vi "Write DI-B Profiles.vi"(8 "error in (no error)":errorcluster, 10 "DI-B Profiles - Pulse Width [s]":sgl[][](array[numeric]), 11 "DCM-DSI-HW in":refnum<class "DCM-DSI.lvclass">) -> (0 "error out":errorcluster, 3 "DCM-DSI-HW out":refnum<class "DCM-DSI.lvclass">)   [LabVIEW 2016, in "DCM-DSI.lvclass"]
uses:
  DCM-DSI.lvclass
  DCM-DSI.lvclass/DCM-DSI.ctl
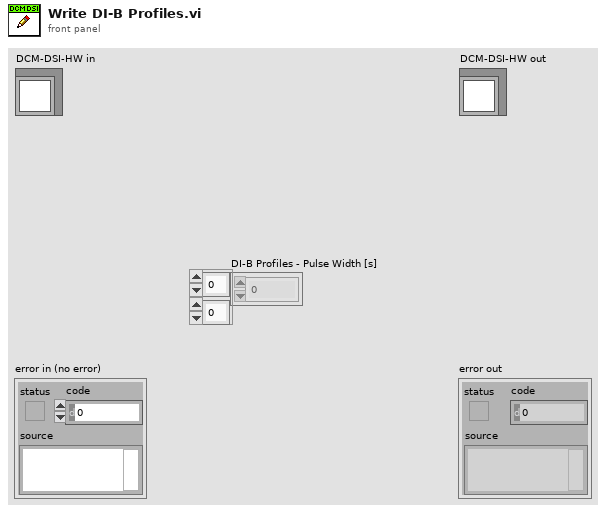
[diagram p1: front panel]
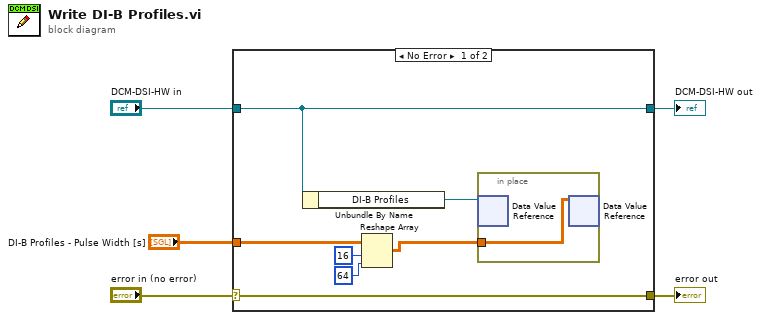
[diagram p0: block diagram]
diagram:
  n1 = case shown="No Error" "error in (no error)" {
    selector: "error in (no error)" -> [w12 w15]
    tunnel: [w12 w15] -> w4
    tunnel: [w10 w14] -> w2
    tunnel: "DCM-DSI-HW in" -> [w10 w14]
    tunnel: "DI-B Profiles - Pulse Width [s]" -> [w7 _]
    frame No Error {
      n2 = Unbundle By Name(w10) -> ("DI-B Profiles"=w11:refnum<data-value>)
      n3 = Reshape Array(w7, 16 ("dimension size"), 64 ("dimension size")) -> (w6:sgl[][])
      n4 = in-place {
        in-place-border: w6 -> [w13]
        n5 = in-place-dvr #1(w11) -> ()  [unwired: 2 out]
        n6 = in-place-dvr #1(w13) -> ()  [unwired: 2 out]
      }
    }
    frame Error {
    }
  }
  "error out" <- w4
  "DCM-DSI-HW out" <- w2
